vi "Shapes.vi"() -> ()   [LabVIEW 2011]
uses:
  <vilib>/Heliosphere Research LLC/Advanced Plotting Toolkit/Advanced Plotting Toolkit.lvlib
  <vilib>/Heliosphere Research LLC/Advanced Plotting Toolkit/typedefs/PlotColor.ctl
  <vilib>/Heliosphere Research LLC/Advanced Plotting Toolkit/properties/Line_Style.ctl
  <vilib>/Heliosphere Research LLC/Advanced Plotting Toolkit/properties/Line.ctl
  <vilib>/Heliosphere Research LLC/Advanced Plotting Toolkit/properties/Display.ctl
  <vilib>/Heliosphere Research LLC/Advanced Plotting Toolkit/api_annotations/ShapeProperties.ctl
panel:
  in  "Y Position":dbl=-1.0 format="%#_13g"
  in  "Height":dbl=2.0 format="%#_13g"
  in  "Z Order":dbl=1.0
  in  "Width":dbl=6.28
  in  "X Position":dbl=3.14 format="%#_13g"
  out "Shapes Demo":picture
  # "Shapes"
  # "It's sometimes useful to highlight a particular region of data\non a plot.  Rectangle.vi and Circle.vi provide a simple\nmechanism for this, by drawing a rectangle or circle on the\nplot at the desired location.\n\nIn this example, a rectangle is used to highlight one cycle of\na sine wave.  Try changing the dimensions, below.\n\nYou can also adjust the Z order, to place the shape behind\nor in front of features on the plot.  Try setting Z Order to 2.\n\nNote that the values used for the position and size of the\nshape are in data units.  This means they are measured using\nthe plot axes, as opposed to an absolute unit like pixels or\npoints."
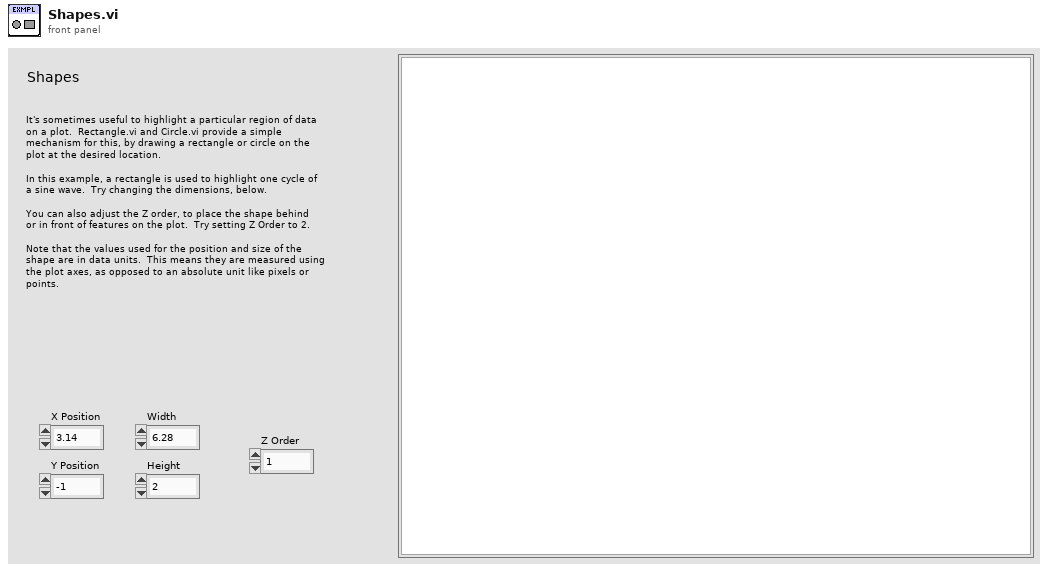
[diagram p1: front panel]
types:
  T1 = typedef "Advanced Plotting Toolkit.lvlib/ShapeProperties.ctl" = cluster{"Color":T2, "Line":T3, "Display":T5}
  T2 = typedef "Advanced Plotting Toolkit.lvlib/PlotColor.ctl" = u32
  T3 = typedef "Advanced Plotting Toolkit.lvlib/Line.ctl" = cluster{"Style":T4, "Color":T2, "Width":sgl}
  T4 = typedef "Advanced Plotting Toolkit.lvlib/Line_Style.ctl" = enum16{"Automatic", "Solid", "Dashed", "Dotted", "Dash-dot", "Invisible"}
  T5 = typedef "Advanced Plotting Toolkit.lvlib/Display.ctl" = cluster{"Alpha":dbl, "Z Order":dbl}
  T6 = typedef "Advanced Plotting Toolkit.lvlib/PlotID.ctl" = i32
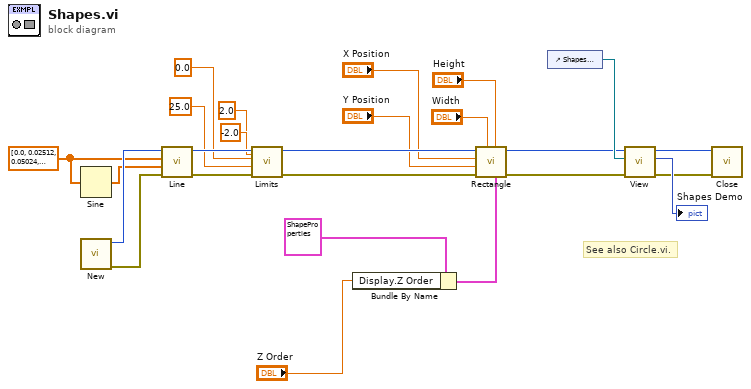
[diagram p0: block diagram]
diagram:
  w11 = dbl[] [0.0, 0.02512, 0.05024, 0.07536000000000001, 0.10048, 0.12560000000000002, 0.15072000000000002, 0.17584000000000002, 0.20096, 0.22608, 0.25120000000000003, 0.27632, 0.30144000000000004, 0.32656, 0.35168000000000005, 0.3768, 0.40192, 0.42704000000000003, 0.45216, 0.47728, 0.5024000000000001, 0.5275200000000001, 0.55264, 0.57776, 0.6028800000000001, 0.6280000000000001, 0.65312, 0.6782400000000001, 0.7033600000000001, 0.72848, 0.7536, 0.7787200000000001, 0.80384, 0.82896, 0.8540800000000001, 0.8792000000000001, 0.90432, 0.92944, 0.95456, 0.97968, 1.0048000000000001, 1.0299200000000002, 1.0550400000000002, 1.08016, 1.10528, 1.1304, 1.15552, 1.1806400000000001, 1.2057600000000002, 1.2308800000000002, 1.2560000000000002, 1.28112, 1.30624, 1.33136, 1.3564800000000001, 1.3816000000000002, 1.4067200000000002, 1.43184, 1.45696, 1.48208, 1.5072, 1.5323200000000001, 1.5574400000000002, 1.58256, 1.60768, 1.6328, 1.65792, 1.68304, 1.7081600000000001, 1.7332800000000002, 1.7584000000000002, 1.78352, 1.80864, 1.83376, 1.85888, 1.884, 1.90912, 1.93424, 1.95936, 1.98448, 2.0096000000000003, 2.03472, 2.0598400000000003, 2.08496, 2.1100800000000004, 2.1352, 2.16032, 2.18544, 2.21056, 2.23568, 2.2608, 2.28592, 2.31104, 2.33616, 2.3612800000000003, 2.3864, 2.4115200000000003, 2.43664, 2.4617600000000004, 2.48688, 2.5120000000000005, 2.5371200000000003, 2.56224, 2.58736, 2.61248, 2.6376, 2.66272, 2.68784, 2.7129600000000003, 2.73808, 2.7632000000000003, 2.78832, 2.8134400000000004, 2.83856, 2.86368, 2.8888000000000003, 2.91392, 2.9390400000000003, 2.96416, 2.98928, 3.0144, 3.03952, 3.0646400000000003, 3.08976, 3.1148800000000003, 3.14, 3.16512, 3.19024, 3.21536, 3.2404800000000002, 3.2656, 3.2907200000000003, 3.31584, 3.3409600000000004, 3.36608, 3.3912000000000004, 3.4163200000000002, 3.4414400000000005, 3.4665600000000003, 3.4916800000000006, 3.5168000000000004, 3.5419199999999997, 3.56704, 3.59216, 3.61728, 3.6424, 3.66752, 3.69264, 3.71776, 3.74288, 3.768, 3.79312, 3.81824, 3.84336, 3.86848, 3.8936, 3.91872, 3.9438400000000002, 3.96896, 3.9940800000000003, 4.0192000000000005, 4.04432, 4.06944, 4.09456, 4.119680000000001, 4.1448, 4.16992, 4.1950400000000005, 4.220160000000001, 4.24528, 4.2704, 4.295520000000001, 4.32064, 4.34576, 4.37088, 4.396, 4.42112, 4.4462399999999995, 4.47136, 4.49648, 4.5216, 4.54672, 4.57184, 4.59696, 4.62208, 4.6472, 4.67232, 4.69744, 4.7225600000000005, 4.74768, 4.7728, 4.79792, 4.823040000000001, 4.84816, 4.87328, 4.8984000000000005, 4.923520000000001, 4.94864, 4.97376, 4.998880000000001, 5.024000000000001, 5.04912, 5.0742400000000005, 5.099360000000001, 5.12448, 5.1495999999999995, 5.17472, 5.19984, 5.22496, 5.25008, 5.2752, 5.30032, 5.32544, 5.35056, 5.37568, 5.4008, 5.4259200000000005, 5.45104, 5.47616, 5.50128, 5.526400000000001, 5.55152, 5.57664, 5.6017600000000005, 5.626880000000001, 5.652, 5.67712, 5.702240000000001, 5.72736, 5.75248, 5.7776000000000005, 5.802720000000001, 5.82784, 5.85296, 5.878080000000001, 5.9032, 5.92832, 5.95344, 5.97856, 6.00368, 6.0288, 6.05392, 6.07904, 6.10416, 6.1292800000000005, 6.1544, 6.17952, 6.20464, 6.229760000000001, 6.25488, 6.28, 6.3051200000000005, 6.33024, 6.35536, 6.38048, 6.405600000000001, 6.43072, 6.45584, 6.4809600000000005, 6.506080000000001, 6.5312, 6.55632, 6.581440000000001, 6.606560000000001, 6.63168, 6.6568000000000005, 6.681920000000001, 6.707040000000001, 6.73216, 6.757280000000001, 6.782400000000001, 6.807520000000001, 6.8326400000000005, 6.857760000000001, 6.882880000000001, 6.908000000000001, 6.933120000000001, 6.958240000000001, 6.983360000000001, 7.0084800000000005, 7.033600000000001, 7.058720000000001, 7.0838399999999995, 7.10896, 7.13408, 7.159199999999999, 7.18432, 7.20944, 7.23456, 7.2596799999999995, 7.2848, 7.30992, 7.33504, 7.36016, 7.38528, 7.4104, 7.43552, 7.46064, 7.48576, 7.51088, 7.536, 7.56112, 7.58624, 7.61136, 7.63648, 7.6616, 7.68672, 7.7118400000000005, 7.73696, 7.76208, 7.7872, 7.812320000000001, 7.83744, 7.86256, 7.8876800000000005, 7.912800000000001, 7.93792, 7.96304, 7.988160000000001, 8.01328, 8.038400000000001, 8.06352, 8.08864, 8.113760000000001, 8.13888, 8.164000000000001, 8.18912, 8.21424, 8.239360000000001, 8.26448, 8.2896, 8.314720000000001, 8.33984, 8.36496, 8.390080000000001, 8.4152, 8.440320000000002, 8.465440000000001, 8.49056, 8.515680000000001, 8.5408, 8.56592, 8.591040000000001, 8.61616, 8.64128, 8.6664, 8.69152, 8.71664, 8.74176, 8.76688, 8.792, 8.81712, 8.84224, 8.86736, 8.892479999999999, 8.9176, 8.94272, 8.96784, 8.99296, 9.01808, 9.0432, 9.06832, 9.09344, 9.11856, 9.14368, 9.168800000000001, 9.19392, 9.21904, 9.24416, 9.26928, 9.2944, 9.31952, 9.34464, 9.369760000000001, 9.39488, 9.42, 9.445120000000001, 9.47024, 9.49536, 9.520480000000001, 9.5456, 9.57072, 9.59584, 9.62096, 9.646080000000001, 9.6712, 9.69632, 9.721440000000001, 9.74656, 9.77168, 9.796800000000001, 9.82192, 9.847040000000002, 9.872160000000001, 9.89728, 9.922400000000001, 9.94752, 9.97264, 9.997760000000001, 10.02288, 10.048000000000002, 10.073120000000001, 10.09824, 10.123360000000002, 10.148480000000001, 10.1736, 10.198720000000002, 10.22384, 10.24896, 10.27408, 10.299199999999999, 10.32432, 10.34944, 10.37456, 10.39968, 10.4248, 10.44992, 10.47504, 10.50016, 10.52528, 10.5504, 10.575520000000001, 10.60064, 10.62576, 10.65088, 10.676, 10.70112, 10.72624, 10.75136, 10.77648, 10.8016, 10.82672, 10.851840000000001, 10.87696, 10.90208, 10.927200000000001, 10.95232, 10.97744, 11.00256, 11.02768, 11.052800000000001, 11.07792, 11.10304, 11.128160000000001, 11.15328, 11.1784, 11.203520000000001, 11.22864, 11.253760000000002, 11.278880000000001, 11.304, 11.329120000000001, 11.35424, 11.37936, 11.404480000000001, 11.4296, 11.45472, 11.479840000000001, 11.50496, 11.530080000000002, 11.555200000000001, 11.58032, 11.605440000000002, 11.630560000000001, 11.65568, 11.680800000000001, 11.70592, 11.731040000000002, 11.756160000000001, 11.78128, 11.8064, 11.83152, 11.85664, 11.88176, 11.90688, 11.932, 11.95712, 11.98224, 12.00736, 12.03248, 12.0576, 12.08272, 12.10784, 12.13296, 12.15808, 12.1832, 12.20832, 12.23344, 12.258560000000001, 12.28368, 12.3088, 12.33392, 12.35904, 12.38416, 12.40928, 12.4344, 12.459520000000001, 12.48464, 12.50976, 12.534880000000001, 12.56, 12.58512, 12.610240000000001, 12.63536, 12.66048, 12.6856, 12.71072, 12.735840000000001, 12.76096, 12.78608, 12.811200000000001, 12.83632, 12.86144, 12.886560000000001, 12.91168, 12.936800000000002, 12.961920000000001, 12.98704, 13.012160000000002, 13.03728, 13.0624, 13.087520000000001, 13.11264, 13.137760000000002, 13.162880000000001, 13.188, 13.213120000000002, 13.238240000000001, 13.26336, 13.288480000000002, 13.313600000000001, 13.33872, 13.363840000000001, 13.38896, 13.414080000000002, 13.439200000000001, 13.46432, 13.489440000000002, 13.514560000000001, 13.53968, 13.564800000000002, 13.589920000000001, 13.615040000000002, 13.640160000000002, 13.665280000000001, 13.690400000000002, 13.715520000000001, 13.74064, 13.765760000000002, 13.790880000000001, 13.816000000000003, 13.841120000000002, 13.866240000000001, 13.891360000000002, 13.916480000000002, 13.941600000000001, 13.966720000000002, 13.991840000000002, 14.016960000000001, 14.042080000000002, 14.067200000000001, 14.092320000000003, 14.117440000000002, 14.14256, 14.167679999999999, 14.1928, 14.21792, 14.243039999999999, 14.26816, 14.29328, 14.318399999999999, 14.34352, 14.36864, 14.393759999999999, 14.41888, 14.443999999999999, 14.46912, 14.49424, 14.519359999999999, 14.54448, 14.5696, 14.594719999999999, 14.61984, 14.64496, 14.67008, 14.6952, 14.72032, 14.74544, 14.77056, 14.795679999999999, 14.8208, 14.84592, 14.87104, 14.89616, 14.92128, 14.9464, 14.97152, 14.99664, 15.02176, 15.04688, 15.072, 15.09712, 15.12224, 15.14736, 15.17248, 15.1976, 15.22272, 15.24784, 15.27296, 15.29808, 15.3232, 15.348320000000001, 15.37344, 15.39856, 15.423680000000001, 15.4488, 15.47392, 15.49904, 15.52416, 15.549280000000001, 15.5744, 15.59952, 15.624640000000001, 15.64976, 15.67488, 15.700000000000001, 15.72512, 15.75024, 15.775360000000001, 15.80048, 15.825600000000001, 15.85072, 15.87584, 15.900960000000001, 15.92608, 15.9512, 15.976320000000001, 16.001440000000002, 16.02656, 16.05168, 16.076800000000002, 16.10192, 16.12704, 16.152160000000002, 16.17728, 16.2024, 16.227520000000002, 16.25264, 16.27776, 16.302880000000002, 16.328000000000003, 16.35312, 16.37824, 16.403360000000003, 16.42848, 16.4536, 16.478720000000003, 16.50384, 16.52896, 16.554080000000003, 16.5792, 16.60432, 16.629440000000002, 16.65456, 16.67968, 16.704800000000002, 16.72992, 16.75504, 16.780160000000002, 16.805280000000003, 16.8304, 16.855520000000002, 16.880640000000003, 16.90576, 16.930880000000002, 16.956000000000003, 16.98112, 17.006240000000002, 17.031360000000003, 17.05648, 17.0816, 17.106720000000003, 17.13184, 17.15696, 17.182080000000003, 17.2072, 17.23232, 17.257440000000003, 17.28256, 17.307679999999998, 17.3328, 17.35792, 17.38304, 17.40816, 17.43328, 17.4584, 17.48352, 17.50864, 17.53376, 17.55888, 17.584, 17.60912, 17.63424, 17.65936, 17.68448, 17.7096, 17.73472, 17.75984, 17.784959999999998, 17.81008, 17.8352, 17.86032, 17.88544, 17.91056, 17.93568, 17.9608, 17.98592, 18.01104, 18.03616, 18.06128, 18.0864, 18.11152, 18.13664, 18.16176, 18.18688, 18.212, 18.23712, 18.26224, 18.28736, 18.31248, 18.337600000000002, 18.36272, 18.38784, 18.41296, 18.43808, 18.4632, 18.48832, 18.51344, 18.53856, 18.56368, 18.5888, 18.61392, 18.63904, 18.66416, 18.68928, 18.7144, 18.739520000000002, 18.76464, 18.78976, 18.814880000000002, 18.84, 18.86512, 18.890240000000002, 18.91536, 18.94048, 18.965600000000002, 18.99072, 19.01584, 19.040960000000002, 19.06608, 19.0912, 19.11632, 19.14144, 19.16656, 19.19168, 19.216800000000003, 19.24192, 19.26704, 19.292160000000003, 19.31728, 19.3424, 19.367520000000003, 19.39264, 19.41776, 19.442880000000002, 19.468, 19.49312, 19.518240000000002, 19.54336, 19.56848, 19.593600000000002, 19.61872, 19.64384, 19.668960000000002, 19.694080000000003, 19.7192, 19.744320000000002, 19.769440000000003, 19.79456, 19.81968, 19.844800000000003, 19.86992, 19.89504, 19.920160000000003, 19.94528, 19.9704, 19.995520000000003, 20.02064, 20.04576, 20.070880000000002, 20.096000000000004, 20.12112, 20.146240000000002, 20.171360000000004, 20.19648, 20.221600000000002, 20.246720000000003, 20.27184, 20.296960000000002, 20.322080000000003, 20.3472, 20.372320000000002, 20.397440000000003, 20.42256, 20.44768, 20.4728, 20.49792, 20.523039999999998, 20.54816, 20.57328, 20.598399999999998, 20.62352, 20.64864, 20.673759999999998, 20.69888, 20.724, 20.74912, 20.77424, 20.79936, 20.82448, 20.8496, 20.87472, 20.89984, 20.92496, 20.95008, 20.9752, 21.00032, 21.02544, 21.05056, 21.07568, 21.1008, 21.12592, 21.151040000000002, 21.17616, 21.20128, 21.2264, 21.25152, 21.27664, 21.30176, 21.32688, 21.352, 21.37712, 21.40224, 21.42736, 21.45248, 21.4776, 21.50272, 21.52784, 21.55296, 21.57808, 21.6032, 21.628320000000002, 21.65344, 21.67856, 21.703680000000002, 21.7288, 21.75392, 21.779040000000002, 21.80416, 21.82928, 21.854400000000002, 21.87952, 21.90464, 21.92976, 21.95488, 21.98, 22.00512, 22.03024, 22.05536, 22.08048, 22.105600000000003, 22.13072, 22.15584, 22.180960000000002, 22.20608, 22.2312, 22.256320000000002, 22.28144, 22.30656, 22.331680000000002, 22.3568, 22.38192, 22.407040000000002, 22.43216, 22.45728, 22.482400000000002, 22.507520000000003, 22.53264, 22.557760000000002, 22.582880000000003, 22.608, 22.63312, 22.658240000000003, 22.68336, 22.70848, 22.733600000000003, 22.75872, 22.78384, 22.808960000000003, 22.83408, 22.8592, 22.884320000000002, 22.90944, 22.93456, 22.959680000000002, 22.984800000000003, 23.00992, 23.035040000000002, 23.060160000000003, 23.08528, 23.110400000000002, 23.135520000000003, 23.16064, 23.185760000000002, 23.210880000000003, 23.236, 23.261120000000002, 23.286240000000003, 23.31136, 23.33648, 23.361600000000003, 23.386720000000004, 23.41184, 23.436960000000003, 23.462080000000004, 23.4872, 23.512320000000003, 23.537440000000004, 23.56256, 23.58768, 23.6128, 23.63792, 23.66304, 23.68816, 23.71328, 23.7384, 23.76352, 23.78864, 23.81376, 23.83888, 23.864, 23.88912, 23.91424, 23.93936, 23.96448, 23.9896, 24.01472, 24.03984, 24.06496, 24.09008, 24.1152, 24.14032, 24.16544, 24.19056, 24.21568, 24.2408, 24.26592, 24.29104, 24.31616, 24.34128, 24.3664, 24.39152, 24.41664, 24.44176, 24.46688, 24.492, 24.517120000000002, 24.54224, 24.56736, 24.592480000000002, 24.6176, 24.64272, 24.66784, 24.69296, 24.71808, 24.7432, 24.76832, 24.79344, 24.81856, 24.84368, 24.8688, 24.89392, 24.919040000000003, 24.94416, 24.96928, 24.994400000000002, 25.01952, 25.04464, 25.069760000000002, 25.09488] ("x*y")
  # "See also Circle.vi."
  n1 = Sine(x=w11) -> (sin(x)=w12:dbl[])
  n2 = call <vilib>:"New.vi"() -> ("error out"=w21:errorcluster, "Plot ID"=w22:T6)  [unwired: 10 in]
  n3 = call <vilib>:"Line.vi"("error in (no error)"=w21, "Y Data"=w12, "X Data"=w11, "Plot ID"=w22) -> ("error out"=w19:errorcluster, "Plot ID out"=w20:T6)  [unwired: 6 in]
  n4 = call <vilib>:"Limits.vi"("Y Max"=2.0, "Y Min"=-2.0, "error in (no error)"=w19, "X Max"=25.0, "X Min"=0.0, "Plot ID"=w20) -> ("error out"=w3:errorcluster, "Plot ID Out"=w16:T6)  [unwired: 4 in]
  n5 = Bundle By Name(cluster=T1 {"Color"=2147483647, "Line"={"Style"=enum."Automatic", "Color"=2147483647, "Width"=nan}, "Display"={"Alpha"=nan, "Z Order"=nan}} ("Shape Properties"), "Display.Z Order"="Z Order") -> (w5:T1)
  n6 = call <vilib>:"Rectangle.vi"("Properties"=w5, "Height"="Height", "Width"="Width", "error in (no error)"=w3, "Y Position"="Y Position", "X Position"="X Position", "Plot ID"=w16) -> ("error out"=w2:errorcluster, "Plot ID Out"=w15:T6)  [unwired: 3 in]
  n7 = control-ref of="Shapes Demo"() -> (w25:refnum<vi>)
  n8 = call <vilib>:"View.vi"("error in (no error)"=w2, "Ref for Sizing"=w25, "Plot ID"=w15) -> ("error out"=w1:errorcluster, "Picture"=→"Shapes Demo":picture, "Plot ID Out"=w23:T6)  [unwired: 6 in]
  n9 = call <vilib>:"Close.vi"("error in (no error)"=w1, "Plot ID"=w23) -> ()  [unwired: 9 in, 1 out]
